vi "Modified Axis Code.vi"() -> ()   [LabVIEW 2015]
uses:
  <vilib>/Platform/TimedLoop/XDataNode/wakeup.ctl
  <vilib>/Platform/TimedLoop/XDataNode/XDNodeRunTimeDep.lvlib
  <vilib>/Platform/TimedLoop/XDataNode/nitl_modes.ctl
  <vilib>/Platform/TimedLoop/XDataNode/timing_clust.ctl
  <vilib>/Platform/TimedLoop/XDataNode/XDataNode.xnode
  <vilib>/rvi/Analysis/measure/butterworth/XNode/niFpgaButterworthFilter.xnode
panel:
  in  "Cluster":cluster{}
  in  "reset":bool
  in  "apos":i32
  in  "Y Reset":bool
  out "Y limit pulse":bool
  out "Y in limit seeking":bool
  out "Y I Setpoint":fxp<+/-,20,3> caption="current setpoint"
  out "Y PWM duty cycles":T1
  out "Y q current error":fxp<+/-,16,4> format="%#.16g"
  out "Y d current error":fxp<+/-,16,4> caption="current error" format="%.21g"
  in  "Y I gains":cluster{"kp":fxp<+,25,7>, "ki":fxp<+,25,7>}={"kp"=0.19964599609375, "ki"=0.06343460083007812}
  in  "Y motor phasing":bool
  in  "Y motor init reset":bool
  out "Y phasing done":bool
  out "Y i2t over current":bool
  in  "Y seeking i2t threshold":fxp<+,18,2>=0.016998291015625
  in  "Y seeking i2t limit":fxp<+,32,20>=2000.0
  out "Y init encoder":i32
  out "Y Actual init Pos (phasing)":i32
  in  "Y Bypass phasing":bool
  in  "Y Actual init Pos (tested AVE)":i32=236461
  in  "Y start e angle":fxp<+,32,1>=1.5
  in  "Y target e angle":fxp<+,32,1>=1.6000000000931323
  out "Y ADC Trigger":bool caption="trigger"
  in  "Y Coil Reverse":bool=TRUE
  out "Y index Position (ENC)":i32 caption="captured position"
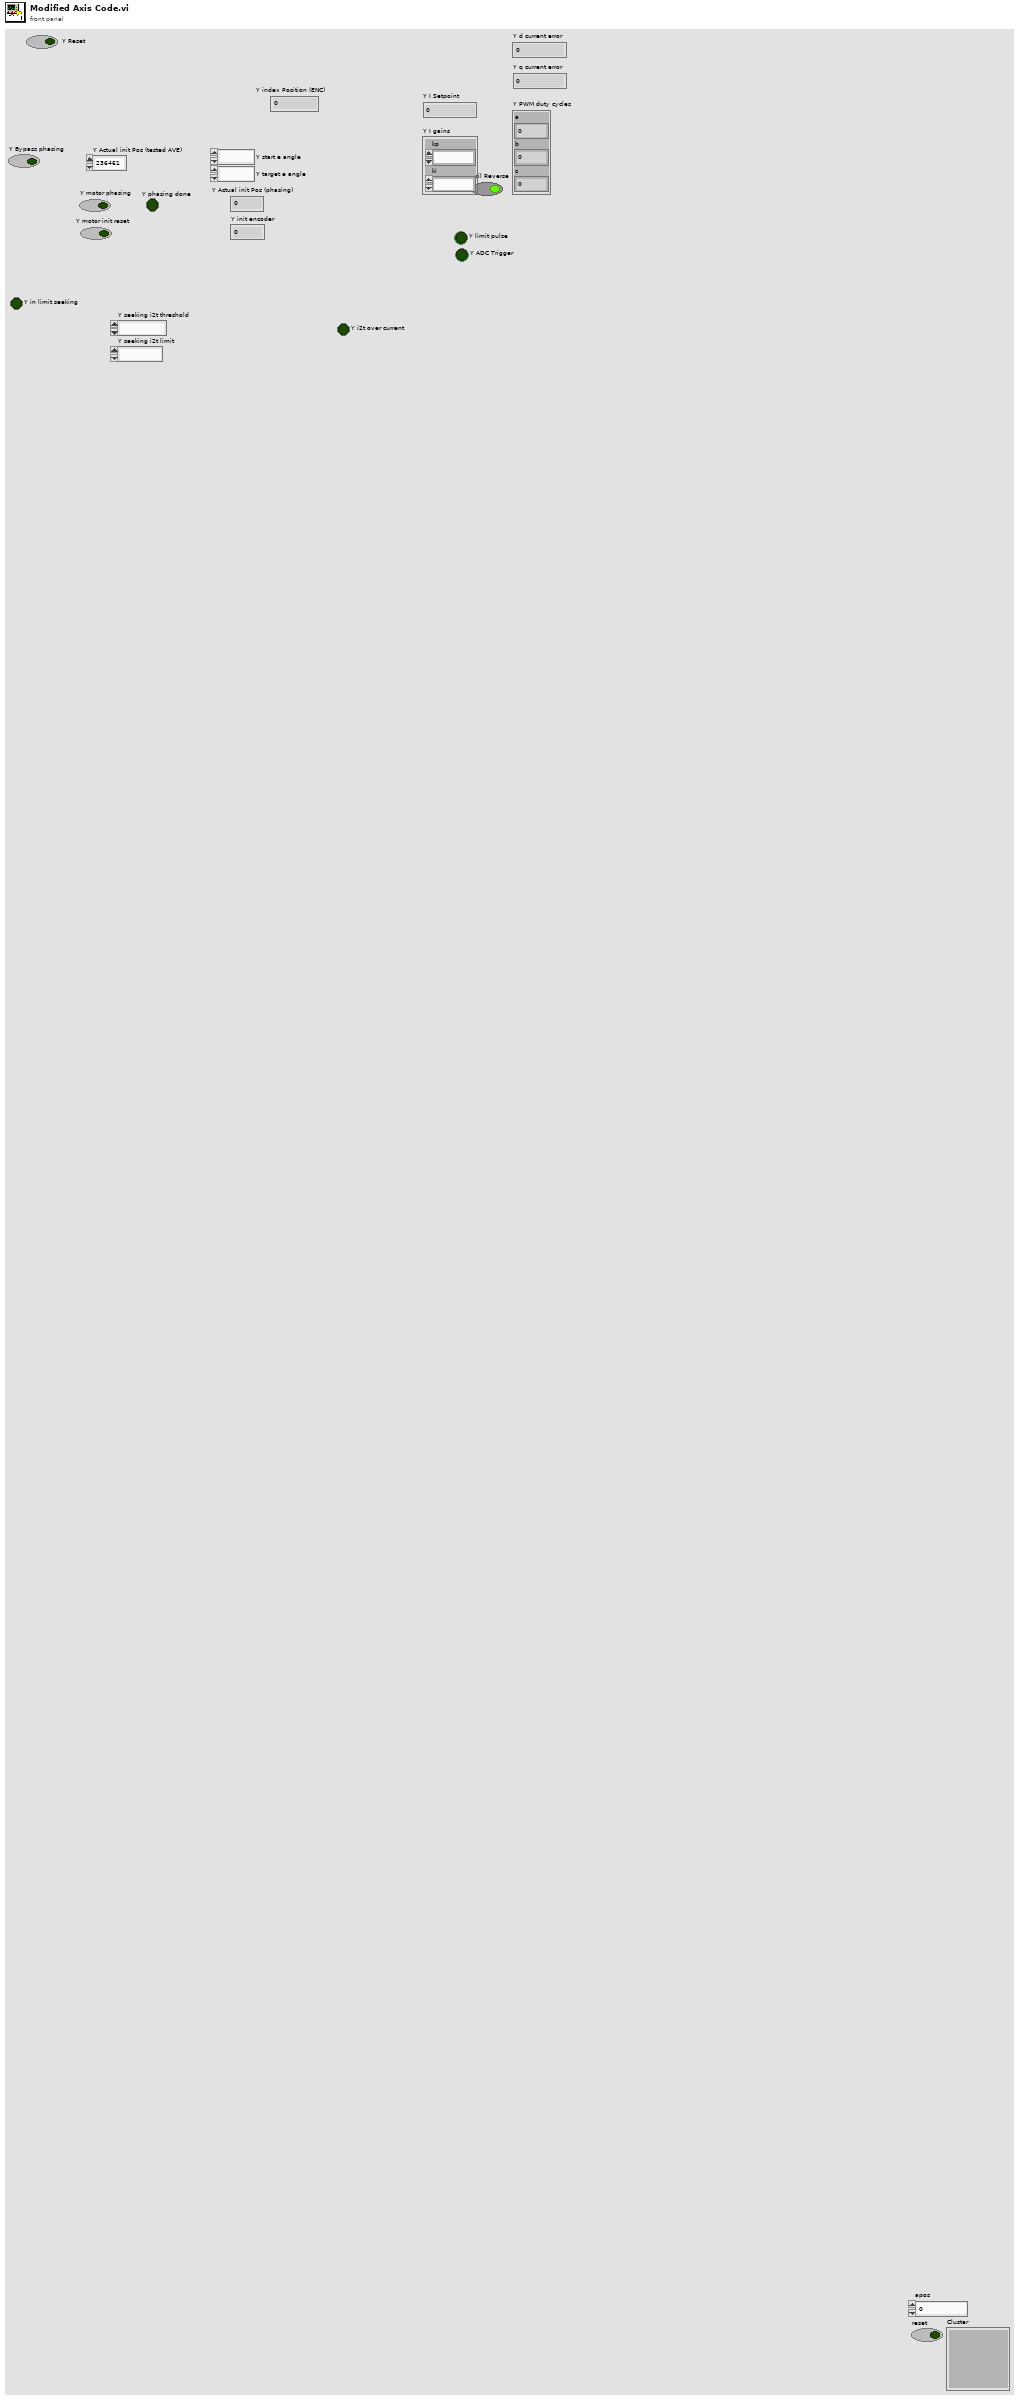
[diagram p1: front panel]
types:
  T1 = cluster{"a":fxp<+,16,1>, "b":fxp<+,16,1>, "c":fxp<+,16,1>}
  T2 = typedef "XDNodeRunTimeDep.lvlib/timing_clust.ctl" = cluster{"Expected End [f-1]":u64, "Actual End [f-1]":u64, "Finished Late? [f-1]":bool, "Expected End [i-1]":u64, "Actual End [i-1]":u64, "Finished Late? [i-1]":bool, "Expected Start [i]":u64, "Actual Start [i]":u64, "Expected Start [f]":u64, "Actual Start [f]":u64, "Source Name":string, "Structure Name":string, "Period":i64, "Deadline":i64, "Offset":i64, "Start":i64, "Priority":i32, "Timeout":i32, "Mode":T3, "Wakeup Reason":T4, "Error":errorcluster, "Source Type":string, "Secondary Source Type":string, "Global End Time":u64, "Global Start Time":u64, "Frame Duration":u64, "Iteration Duration":u64, "Assigned CPU":i32, "I/O Scan Engine Mode":u32}
  T3 = typedef "XDNodeRunTimeDep.lvlib/nitl_modes.ctl" = enum32{"No Change", "Process missed periods, maintain original phase", "Discard missed periods, maintain original phase", "Process missed periods, ignore original phase", "Discard missed periods, ignore original phase"}
  T4 = typedef "XDNodeRunTimeDep.lvlib/wakeup.ctl" = enum32{"Normal", "Aborted", "Asynchronous wakeup", "Timing source error", "Timed loop error", "Timeout"}
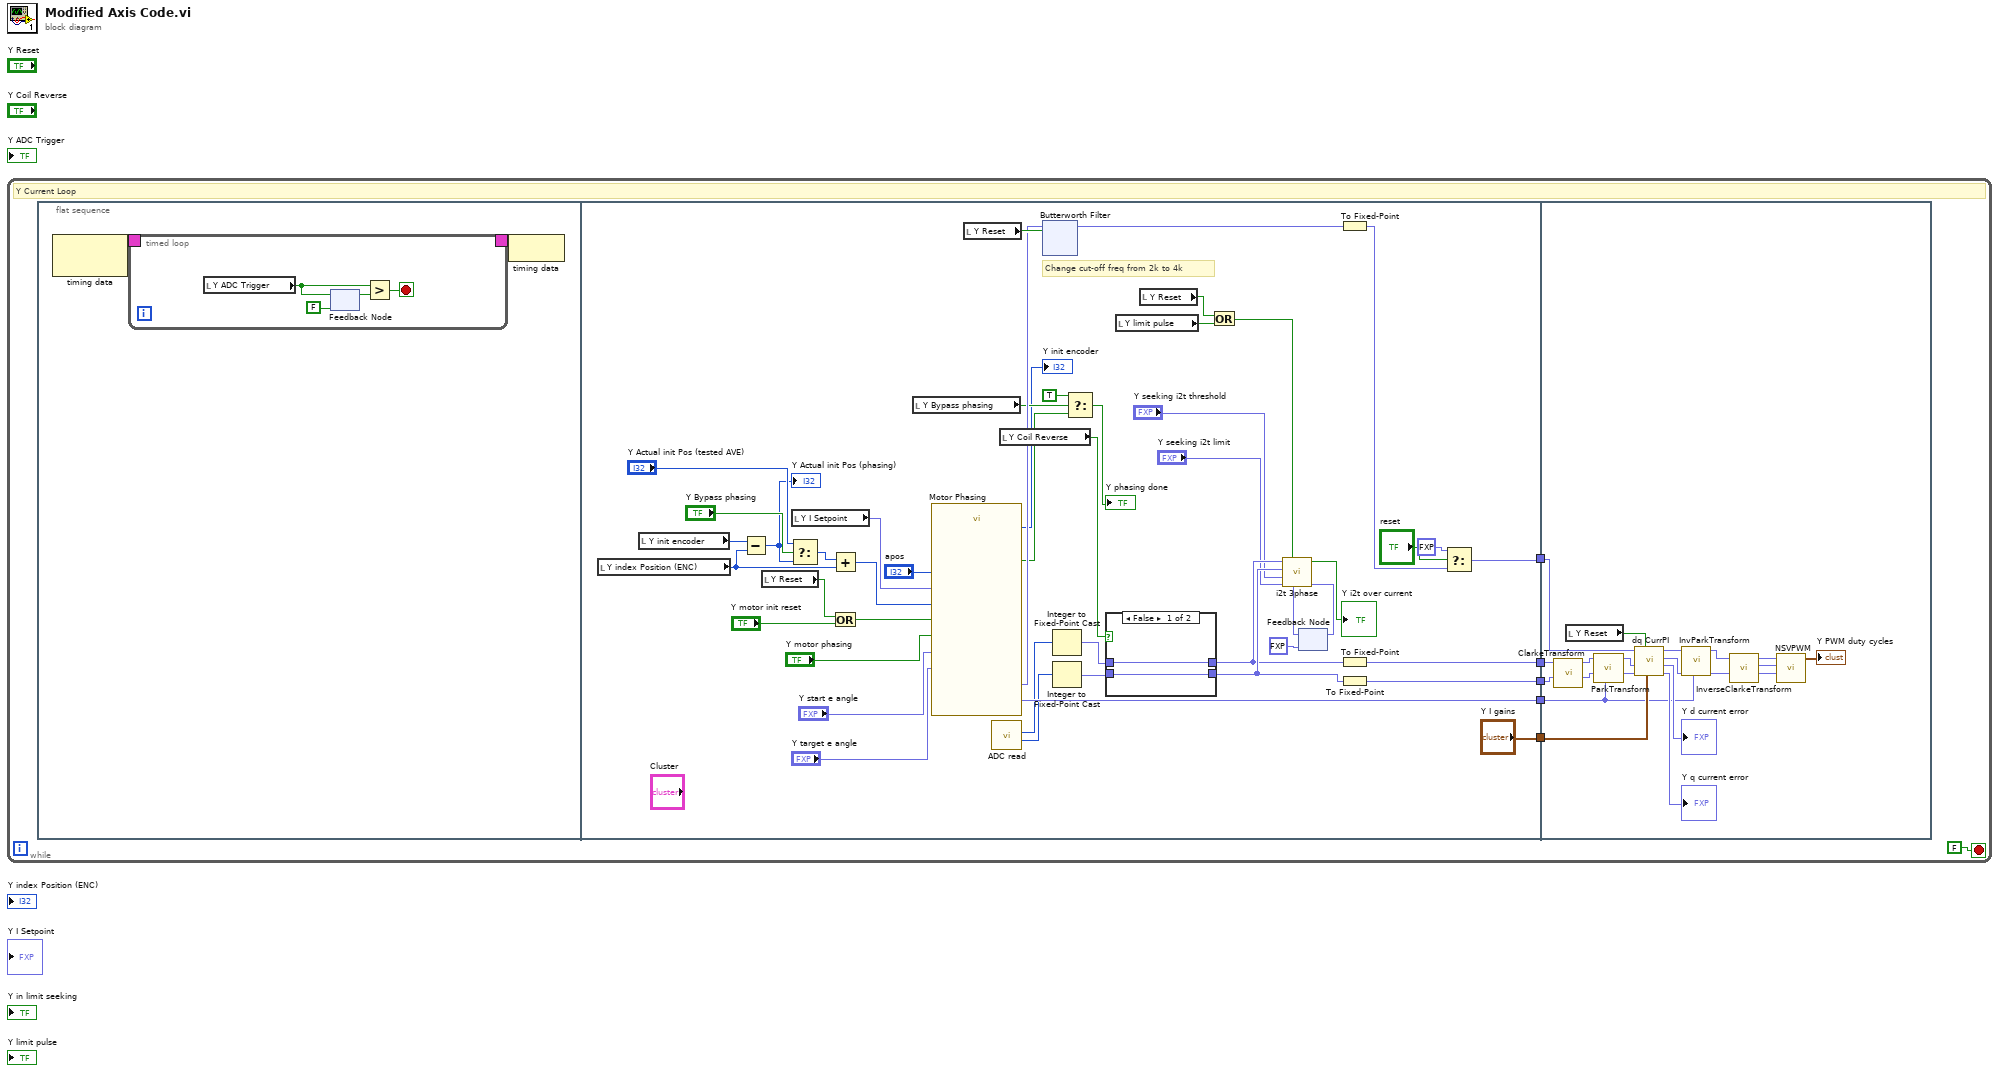
[diagram p0: block diagram]
diagram:
  n1 = while {
    stop <- FALSE stop-if-true
    # "Y Current Loop"
    n2 = flat-sequence {
      tunnel: ["Y I gains"] -> w5
      tunnel: [w58] -> w4
      tunnel: [w59] -> w3
      tunnel: [w42] -> w2
      tunnel: [w46] -> w1
      tunnel: w5 -> [w88]
      tunnel: w4 -> [w85]
      tunnel: w3 -> [w84]
      tunnel: w2 -> [w76]
      tunnel: w1 -> [w87]
      frame #0 {
        n3 = node-c288() -> (w8:T2)  [unwired: 1 in]
        n4 = timed-loop {
          timing: w8 -> [_]
          timing-out: [_] -> w7
          stop <- w9 stop-if-true
          n5 = local read "Y ADC Trigger"() -> (w10:bool)
          n6 = feedback #1(FALSE ("ADC conv")) -> (w12:bool)
          n7 = feedback-in #1(w10) -> ()
          n8 = Greater?(x=w10, y=w12) -> (0:w9:bool)
        }
        n9 = node-c288(w7) -> ()
      }
      frame #1 {
        # "Change cut-off freq from 2k to 4k"
        n10 = local read "Y index Position (ENC)"() -> (w31:i32)
        n11 = local read "Y init encoder"() -> (w30:i32)
        n12 = Subtract(x=w30, y=w31) -> (x-y=w33:i32)
        "Y Actual init Pos (phasing)" <- w33
        n13 = local read "Y Reset"() -> (w56:bool)
        n14 = Select(t="Y Actual init Pos (tested AVE)", s="Y Bypass phasing", f=w33) -> (s? t:f=w32:i32)
        n15 = local read "Y I Setpoint"() -> (w43:fxp<+/-,20,3>)
        n16 = Add(x=w32, y=w31) -> (x+y=w25:i32)
        n17 = Or(x=w56, y="Y motor init reset") -> (x .or. y?=w45:bool)
        n18 = local read "Y Bypass phasing"() -> (w27:bool)
        n19 = call "Motor Phasing.vi"("target e angle"="Y target e angle", "start e angle"="Y start e angle", "motor reset"=w45, "init encoder in"=w25, "apos"="apos", "current reference"=w43, "phasing"="Y motor phasing") -> ("phasing done"=w24:bool, "electrical angle"=w42:fxp<+,32,1>, "init encoder"=→"Y init encoder":i32, "current setpoint"=w41:fxp<+/-,20,3>)  [unwired: 1 in]
        n20 = local read "Y Reset"() -> (w55:bool)
        n21 = call "ADC read.vi"() -> ("ADC1"=w19:i16, "ADC0"=w20:i16)  [unwired: 10 in]
        n22 = local read "Y Coil Reverse"() -> (w62:bool)
        n23 = xnode "Butterworth Filter"("input data"=w41, "reset"=w55) -> ("output data"=w53:fxp<+/-,24,7>)  [unwired: 1 in]
        n24 = Integer to Fixed-Point Cast(integer=w20) -> (fixed-point=w61:fxp<+/-,16,1>)  [unwired: 1 in]
        n25 = Integer to Fixed-Point Cast(integer=w19) -> (fixed-point=w60:fxp<+/-,16,1>)  [unwired: 1 in]
        n26 = Select(t=TRUE, s=w27, f=w24) -> (s? t:f=→"Y phasing done":bool)
        n27 = case shown="False" w62 {
          tunnel: w61 -> [w73 w74]
          tunnel: [w73 w75] -> w49
          tunnel: w60 -> [w72 w75]
          tunnel: [w72 w74] -> w50
          frame False {
          }
          frame True {
          }
        }
        n28 = local read "Y limit pulse"() -> (w29:bool)
        n29 = local read "Y Reset"() -> (w37:bool)
        n30 = Or(x=w37, y=w29) -> (x .or. y?=w36:bool)
        n31 = feedback #2(fxp<+,32,20> 0.0 ("i curr2")) -> (w40:fxp<+,32,20>)
        n32 = call "i2t 3phase.vi"("prv i curr2"=w40, "reset"=w36, "limit"="Y seeking i2t limit", "threshold"="Y seeking i2t threshold", "curr C"=w50, "curr A"=w49) -> ("i curr2"=w51:fxp<+,32,20>, "i2t over current"=→"Y i2t over current":bool)  [unwired: 4 in]
        n33 = feedback-in #2(w51) -> ()
        n34 = To Fixed-Point(number=w53) -> (fixed-point=w48:fxp<+/-,20,3>)  [unwired: 1 in]
        n35 = To Fixed-Point(number=w49) -> (fixed-point=w58:fxp<+/-,18,1>)  [unwired: 1 in]
        n36 = To Fixed-Point(number=w50) -> (fixed-point=w59:fxp<+/-,18,1>)  [unwired: 1 in]
        n37 = Select(t=fxp<+/-,20,3> 0.0, s="reset", f=w48) -> (s? t:f=w46:fxp<+/-,20,3>)
      }
      frame #2 {
        n38 = call "ClarkeTransform.vi"("c current"=w84, "a current"=w85) -> ("beta current"=w86:fxp<+/-,20,2>, "alpha current"=w83:fxp<+/-,20,2>)  [unwired: 8 in]
        n39 = local read "Y Reset"() -> (w77:bool)
        n40 = call "ParkTransform.vi"("electrical angle"=w76, "beta current"=w86, "alpha current"=w83) -> ("quad current"=w78:fxp<+/-,20,3>, "direct current"=w79:fxp<+/-,20,3>)  [unwired: 7 in]
        n41 = call "dq CurrPI.vi"("gains"=w88, "reset"=w77, "quad current"=w78, "direct current"=w79, "current setpoint"=w87) -> ("q current error"=→"Y q current error":fxp<+/-,16,4>, "d current error"=→"Y d current error":fxp<+/-,16,4>, "quad voltage"=w89:fxp<+/-,20,2>, "direct voltage"=w90:fxp<+/-,20,2>)  [unwired: 3 in]
        n42 = call "InvParkTransform.vi"("electrical angle"=w76, "quad voltage"=w89, "direct voltage"=w90) -> ("voltage beta"=w80:fxp<+/-,20,2>, "voltage alpha"=w91:fxp<+/-,20,2>)  [unwired: 7 in]
        n43 = call "InverseClarkeTransform.vi"("beta voltage"=w80, "alpha voltage"=w91) -> ("c voltage"=w92:fxp<+/-,20,2>, "b voltage"=w93:fxp<+/-,20,2>, "a voltage"=w94:fxp<+/-,20,2>)  [unwired: 7 in]
        n44 = call "NSVPWM.vi"("volt c"=w92, "volt b"=w93, "volt a"=w94) -> ("duty cycles"=→"Y PWM duty cycles":T1)  [unwired: 8 in]
      }
    }
  }
